vi "Update Client Data Representation_just_treatment.vi"(8 "error in (no error)":errorcluster, 11 "Control-Client in":refnum<class "Control-Client.lvclass">) -> (0 "error out":errorcluster, 3 "Control-Client out":refnum<class "Control-Client.lvclass">)   [LabVIEW 2015, in "Control-Client.lvclass"]
uses:
  Control-Client.lvclass
  Control-Client.lvclass/Control-Client.ctl
  methods/Read Group #.vi
  Experiments/Experiments_group.lvclass
  Experiments/Experiment.lvclass
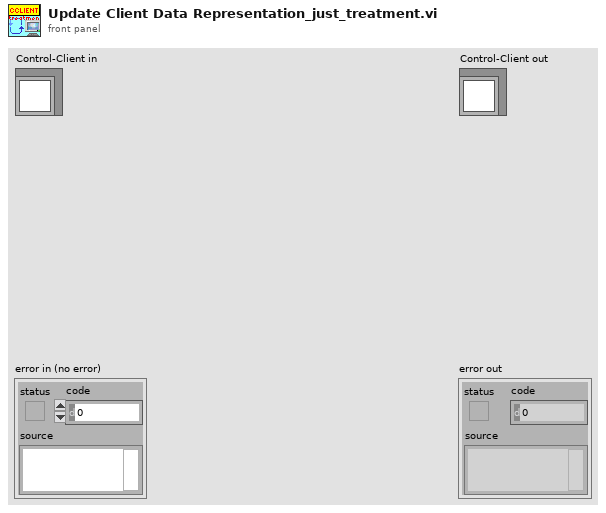
[diagram p1: front panel]
types:
  T1 = typedef "Control-Client.lvclass/Delays-refs_CLIENT.ctl" = cluster{"# points":refnum<vi>, "Step, ps":refnum<vi>, "OZ, ps":refnum<vi>, "# current":refnum<vi>, "RDT, ps":refnum<vi>, "Total length, ps":refnum<vi>, "Kinetics length, ps":refnum<vi>, "Real zero, ps":refnum<vi>, "# par point":refnum<vi>}
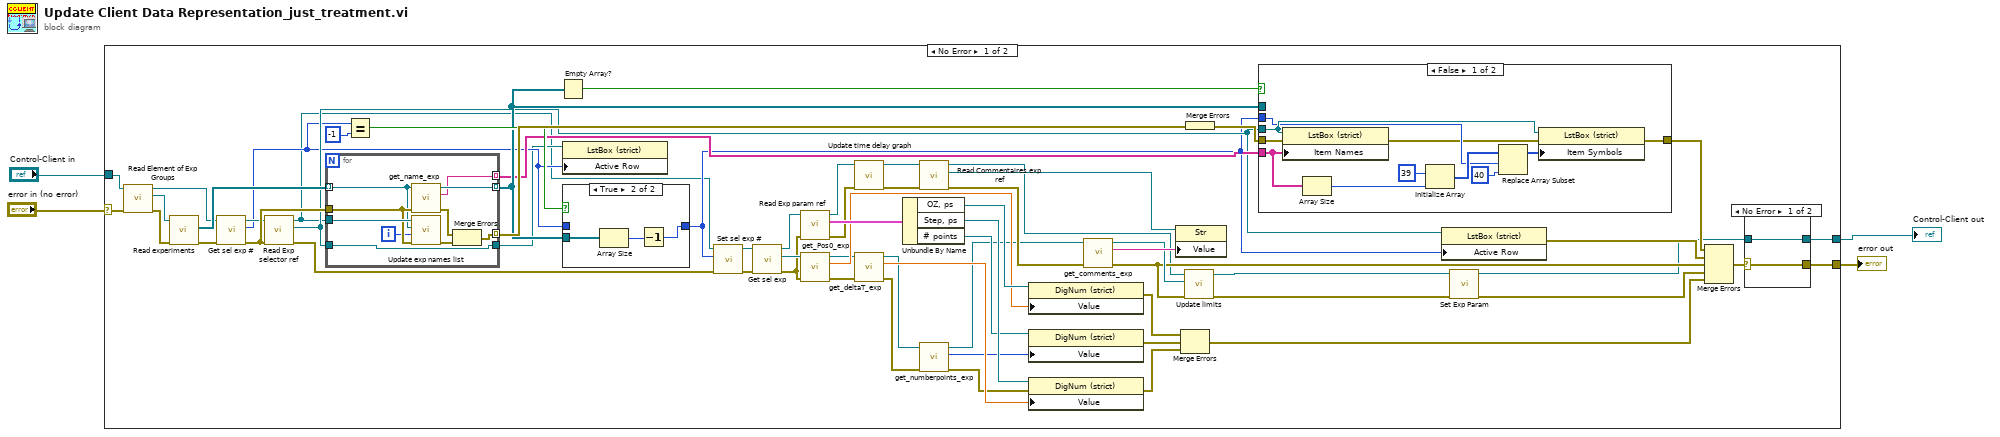
[diagram p0: block diagram]
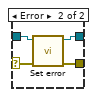
[diagram p2: hidden frame]
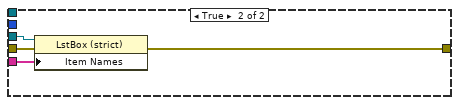
[diagram p4: hidden frame]
diagram:
  n1 = case shown="No Error" "error in (no error)" {
    selector: "error in (no error)" -> [w66 w104]
    tunnel: [w6 w104] -> w3
    tunnel: [w7 w103] -> w1
    tunnel: "Control-Client in" -> [w67 w103]
    frame No Error {
      n2 = call "Read Element of Exp Groups.vi"("error in (no error)"=w66, "Control-Client in"=w67) -> ("error out"=w64:errorcluster, "Experiments_group.lvclass"=w65:refnum<class "Experiments_group.lvclass">, "Control-Client out"=w60:refnum<class "Control-Client.lvclass">)  [unwired: 7 in]
      n3 = call "Read experiments.vi"("error in (no error)"=w64, "Experiments_group.lvclass in"=w65) -> ("error out"=w62:errorcluster, "Experiments"=w63:refnum<class "Experiment.lvclass">[])  [unwired: 6 in, 1 out]
      n4 = call "Get sel exp #.vi"("error in (no error)"=w62, "Control-Client in"=w60) -> ("error out"=w61:errorcluster, "Exp sel #"=w42:i32, "Control-Client out"=w59:refnum<class "Control-Client.lvclass">)  [unwired: 7 in]
      n5 = call "Read Exp selector ref.vi"("error in (no error)"=w61, "Control-Client in"=w59) -> ("error out"=w39:errorcluster, "Exp selector ref"=w43:refnum<vi>, "Control-Client out"=w5:refnum<class "Control-Client.lvclass">)  [unwired: 7 in]
      n6 = for {
        tunnel: w43 -> [w78]
        tunnel: w63 -> [w79] mode=indexing
        tunnel: w5 -> [w87]
        tunnel: w61 -> [w81]
        tunnel: [w84] -> w54 mode=indexing
        tunnel: [w83] -> w50 mode=indexing
        tunnel: [w82] -> w44 mode=indexing
        tunnel: [w78] -> w41
        i -> [w80]
        n7 = call "get_name_exp.vi"("error in (no error)"=w81, "Experiment.lvclass in"=w79) -> ("error out"=w86:errorcluster, "Exp name"=w82:string, "Experiment.lvclass out"=w83:refnum<class "Experiment.lvclass">)  [unwired: 7 in]
        n8 = call "Update exp names list.vi"("error in (no error)"=w81, "# row"=w80, "Experiment in"=w79, "Control-Client in"=w87) -> ("error out"=w85:errorcluster)  [unwired: 6 in, 1 out]
        n9 = Merge Errors(w86, w85) -> (w84:errorcluster)
      }
      n10 = Equal?(x=w42, y=-1) -> (x = y?=w51:bool)
      n11 = Empty Array?(array=w50) -> (empty?=w58:bool)
      n12 = property class="LstBox (strict)"(reference=w41, "Active Row"=w42) -> ()  [unwired: 1 in, 2 out]
      n13 = case shown="True" w51 {
        tunnel: [w74 w75] -> w40
        tunnel: w42 -> [w74 _]
        tunnel: w50 -> [_ w77]
        frame False {
        }
        frame True {
          n14 = Array Size(array=w77) -> (size(s)=w76:i32)
          n15 = Decrement(x=w76) -> (x-1=w75:i32)
        }
      }
      n16 = call "Set sel exp #.vi"("error in (no error)"=w39, "Exp sel #"=w40, "Control-Client in"=w5) -> ("error out"=w24:errorcluster, "Control-Client out"=w22:refnum<class "Control-Client.lvclass">)  [unwired: 7 in]
      n17 = call "Get sel exp.vi"("error in (no error)"=w24, "Control-Client in"=w22) -> ("error out"=w16:errorcluster, "Sel experiment"=w23:refnum<class "Experiment.lvclass">, "Control-Client out"=w21:refnum<class "Control-Client.lvclass">)  [unwired: 7 in]
      n18 = call "Read Exp param ref.vi"("error in (no error)"=w16, "Control-Client in"=w21) -> ("error out"=w20:errorcluster, "Exp param ref"=w36:T1, "Control-Client out"=w19:refnum<class "Control-Client.lvclass">)  [unwired: 7 in]
      n19 = call "get_Pos0_exp.vi"("error in (no error)"=w16, "Experiment.lvclass in"=w23) -> ("error out"=w14:errorcluster, "Delay0,ps"=w34:dbl, "Experiment.lvclass out"=w15:refnum<class "Experiment.lvclass">)  [unwired: 6 in]
      n20 = call "Update time delay graph.vi"("error in (no error)"=w20, "Control-Client en entrée"=w19) -> ("error out"=w18:errorcluster, "Control-Client en sortie"=w17:refnum<class "Control-Client.lvclass">)  [unwired: 8 in]
      n21 = call "get_deltaT_exp.vi"("error in (no error)"=w14, "Experiment.lvclass in"=w15) -> ("error out"=w13:errorcluster, "deltaTlast"=w32:dbl, "Experiment.lvclass out"=w12:refnum<class "Experiment.lvclass">)  [unwired: 7 in]
      n22 = Unbundle By Name(w36) -> ("OZ, ps"=w35:refnum<vi>, "Step, ps"=w33:refnum<vi>, "# points"=w31:refnum<vi>)
      n23 = call "Read Commentaires exp ref.vi"("error in (no error)"=w18, "Control-Client in"=w17) -> ("error out"=w55:errorcluster, "Commentaires exp ref"=w56:refnum<vi>, "Control-Client out"=w45:refnum<class "Control-Client.lvclass">)  [unwired: 7 in]
      n24 = call "get_numberpoints_exp.vi"("error in (no error)"=w13, "Experiment.lvclass in"=w12) -> ("error out"=w26:errorcluster, "numberpoints"=w30:i32, "Experiment.lvclass out"=w11:refnum<class "Experiment.lvclass">)  [unwired: 7 in]
      n25 = property class="DigNum (strict)"(reference=w35, "Value"=w34) -> (error out=w29:errorcluster)  [unwired: 1 in, 1 out]
      n26 = property class="DigNum (strict)"(reference=w31, "Value"=w30) -> (error out=w28:errorcluster)  [unwired: 1 in, 1 out]
      n27 = property class="DigNum (strict)"(reference=w33, error in=w26, "Value"=w32) -> (error out=w27:errorcluster)  [unwired: 1 out]
      n28 = call "get_comments_exp.vi"("error in (no error)"=w55, "Experiment.lvclass in"=w11) -> ("error out"=w46:errorcluster, "Comments"=w57:string, "Experiment.lvclass out"=w47:refnum<class "Experiment.lvclass">)  [unwired: 7 in]
      n29 = property class="Str"(reference=w56, "Value"=w57) -> ()  [unwired: 1 in, 2 out]
      n30 = Merge Errors(w29, w28, w27) -> (w25:errorcluster)
      n31 = call "Update limits.vi"("error in (no error)"=w46, "Experiment.lvclass in"=w47, "Control-Client in"=w45) -> ("error out"=w37:errorcluster, "Control-Client out"=w38:refnum<class "Control-Client.lvclass">)  [unwired: 7 in]
      n32 = Merge Errors(w54) -> (w53:errorcluster)
      n33 = case shown="False" w58 {
        tunnel: w50 -> [_ _]
        tunnel: w43 -> [w93 w102]
        tunnel: w40 -> [w92 _]
        tunnel: w53 -> [w91 w101]
        tunnel: [w89 w100] -> w49
        tunnel: w44 -> [w88 w99]
        frame False {
          n34 = property on="Property Node" class="LstBox (strict)"(reference=w93, error in=w91, "Item Names"=w88) -> (error out=w90:errorcluster)  [unwired: 1 out]
          n35 = Array Size(array=w88) -> (size(s)=w94:i32)
          n36 = Initialize Array(39, w94) -> (w96:i32[])
          n37 = Replace Array Subset(array=w96, new element=40 ("new element/subarray"), index=w92) -> (w95:i32[])
          n38 = property on="Property Node" class="LstBox (strict)"(reference=w93, error in=w90, "Item Symbols"=w95) -> (error out=w89:errorcluster)  [unwired: 1 out]
        }
        frame True {
          n39 = property on="Property Node" class="LstBox (strict)"(reference=w102, error in=w101, "Item Names"=w99) -> (error out=w100:errorcluster)  [unwired: 1 out]
        }
      }
      n40 = property on="Property Node" class="LstBox (strict)"(reference=w43, "Active Row"=w40) -> (error out=w48:errorcluster)  [unwired: 1 in, 1 out]
      n41 = call "Set Exp Param.vi"("Control-Client in"=w38, "error in (no error)"=w37) -> ("Control-Client out"=w9:refnum<class "Control-Client.lvclass">, "error out"=w10:errorcluster)  [unwired: 12 in]
      n42 = Merge Errors(w49, w48, w46, w10, w25) -> (w8:errorcluster)
      n43 = case shown="No Error" w8 {
        selector: w8 -> [w69 w70]
        tunnel: w9 -> [w68 w73]
        tunnel: [w69 w72] -> w6
        tunnel: [w68 w71] -> w7
        frame No Error {
        }
        frame Error {
          n44 = call "Set error.vi"("error in (no error)"=w70, "Control-Client in"=w73) -> ("error out"=w72:errorcluster, "Control-Client out"=w71:refnum<class "Control-Client.lvclass">)  [unwired: 8 in]
        }
      }
    }
    frame Error {
    }
  }
  "error out" <- w3
  "Control-Client out" <- w1
